vi "Initialize.vi"(8 "error in (no error)":errorcluster, 11 "Instrument in":refnum<class "Instrument.lvclass">) -> (0 "error out":errorcluster, 3 "Instrument out":refnum<class "Instrument.lvclass">)   [LabVIEW 2018, in "Instrument.lvclass"]
uses:
  Instrument.lvclass
  C:/Users/observer/Desktop/Sparc4GUI/SPARC4_GUI/Server/Server.lvclass
  Server/Server.lvclass/Server.ctl
  Instrument.lvclass/Instrument.ctl
  Device/Optics/Optics.lvclass/Optics.ctl
  Device/Optics/Opt_Selector/Opt_Selector.lvclass
  C:/Users/observer/Desktop/Sparc4GUI/SPARC4_GUI/Device/Optics/Optics.lvclass
  Device/Optics/Opt_Continuous/Opt_Continuous.lvclass
  Server/Server.lvclass
  Comm/Stream/Stream.lvclass
  Log/Log.lvclass
  StateMachine/State Machine.lvclass
  Device/Optics/Optics.lvclass
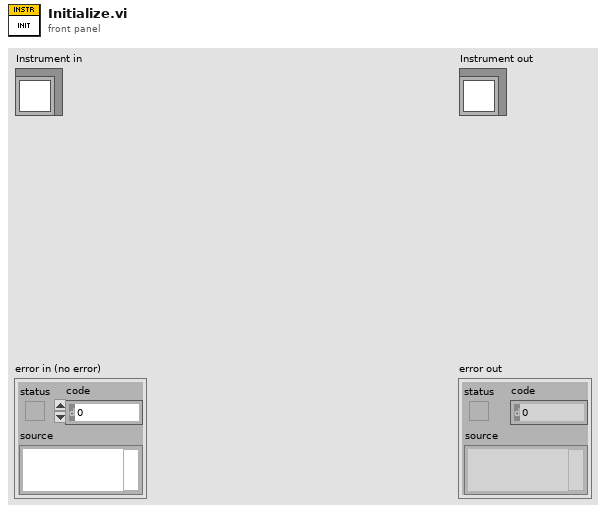
[diagram p1: front panel]
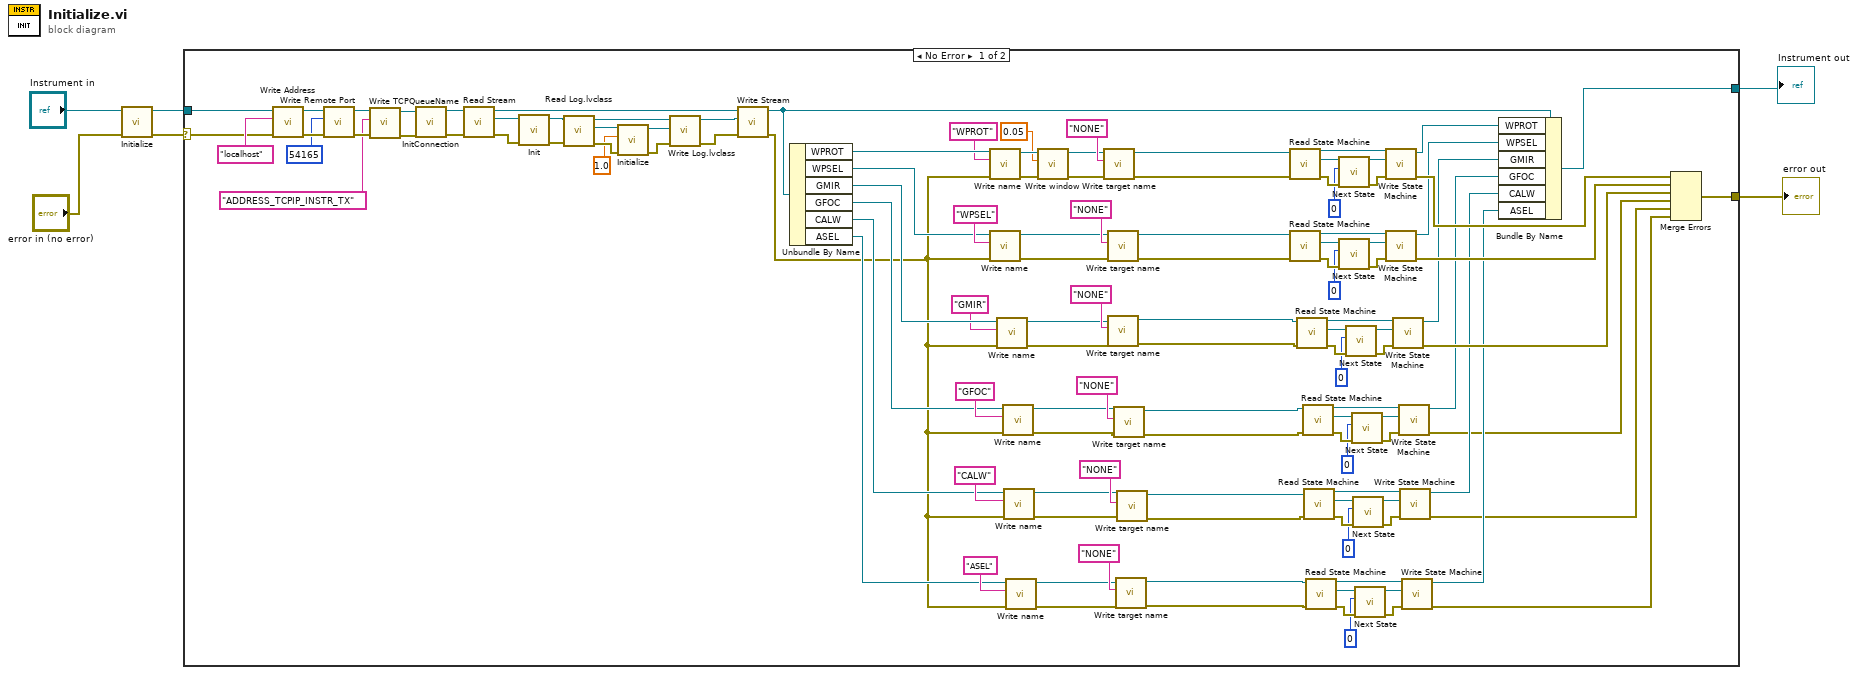
[diagram p0: block diagram]
diagram:
  n1 = call-parent "Initialize.vi"("error in (no error)"="error in (no error)", "Server in"="Instrument in") -> ("error out"=w3:errorcluster, "Server out"=w4:refnum<class "Instrument.lvclass">)  [unwired: 8 in]
  n2 = case shown="No Error" w3 {
    selector: w3 -> [w89 w131]
    tunnel: [w52 w130] -> w1
    tunnel: w4 -> [w90 w130]
    tunnel: [w109 w131] -> w2
    frame No Error {
      n3 = call "Write Address.vi"("error in (no error)"=w89, "Address"="localhost" ("Address:"), "Server in"=w90) -> ("error out"=w93:errorcluster, "Server out"=w94:refnum<class "Instrument.lvclass">)  [unwired: 7 in]
      n4 = call "Write Remote Port.vi"("error in (no error)"=w93, "Remote Port"=u32 54165 ("Remote Port:"), "Server in"=w94) -> ("error out"=w19:errorcluster, "Server out"=w21:refnum<class "Instrument.lvclass">)  [unwired: 7 in]
      n5 = call-dynamic "Write TCPQueueName.vi"("error in (no error)"=w19, "TCPQueueName"="ADDRESS_TCPIP_INSTR_TX", "Server in"=w21) -> ("error out"=w18:errorcluster, "Server out"=w20:refnum<class "Instrument.lvclass">)  [unwired: 7 in]
      n6 = call-dynamic "InitConnection.vi"("error in (no error)"=w18, "Instrument in"=w20) -> ("error out"=w96:errorcluster, "Instrument out"=w95:refnum<class "Instrument.lvclass">)  [unwired: 8 in]
      n7 = call-dynamic "Read Stream.vi"("error in (no error)"=w96, "Server in"=w95) -> ("error out"=w128:errorcluster, "Stream.lvclass"=w53:refnum<class "Stream.lvclass">, "Server out"=w129:refnum<class "Instrument.lvclass">)  [unwired: 7 in]
      n8 = call-dynamic "Init.vi"("error in (no error)"=w128, "Stream in"=w53) -> ("error out"=w10:errorcluster, "Stream out"=w11:refnum<class "Stream.lvclass">)  [unwired: 8 in]
      n9 = call-dynamic "Read Log.lvclass.vi"("error in (no error)"=w10, "Comm in"=w11) -> ("error out"=w13:errorcluster, "Log.lvclass"=w15:refnum<class "Log.lvclass">, "Comm out"=w16:refnum<class "Stream.lvclass">)  [unwired: 7 in]
      n10 = call-dynamic "Initialize.vi"("error in (no error)"=w13, "Level"=1.0, "Log in"=w15) -> ("error out"=w12:errorcluster, "Log out"=w14:refnum<class "Log.lvclass">)  [unwired: 7 in]
      n11 = call-dynamic "Write Log.lvclass.vi"("error in (no error)"=w12, "Log.lvclass"=w14, "Comm in"=w16) -> ("error out"=w8:errorcluster, "Comm out"=w9:refnum<class "Stream.lvclass">)  [unwired: 7 in]
      n12 = call-dynamic "Write Stream.vi"("error in (no error)"=w8, "Stream.lvclass"=w9, "Server in"=w129) -> ("error out"=w63:errorcluster, "Server out"=w54:refnum<class "Instrument.lvclass">)  [unwired: 7 in]
      n13 = Unbundle By Name(w54) -> ("WPROT"=w120:refnum<class "Opt_Selector.lvclass">, "WPSEL"=w111:refnum<class "Opt_Selector.lvclass">, "GMIR"=w100:refnum<class "Opt_Continuous.lvclass">, "GFOC"=w81:refnum<class "Opt_Continuous.lvclass">, "CALW"=w65:refnum<class "Opt_Selector.lvclass">, "ASEL"=w64:refnum<class "Opt_Selector.lvclass">)
      n14 = call-dynamic "Write name.vi"("error in (no error)"=w63, "name"="WPROT", "Optics in"=w120) -> ("error out"=w57:errorcluster, "Optics out"=w56:refnum<class "Opt_Selector.lvclass">)  [unwired: 7 in]
      n15 = call-dynamic "Write name.vi"("error in (no error)"=w63, "name"="WPSEL", "Optics in"=w111) -> ("error out"=w44:errorcluster, "Optics out"=w45:refnum<class "Opt_Selector.lvclass">)  [unwired: 7 in]
      n16 = call-dynamic "Write name.vi"("error in (no error)"=w63, "name"="GMIR", "Optics in"=w100) -> ("error out"=w35:errorcluster, "Optics out"=w37:refnum<class "Opt_Continuous.lvclass">)  [unwired: 7 in]
      n17 = call-dynamic "Write name.vi"("error in (no error)"=w63, "name"="GFOC", "Optics in"=w81) -> ("error out"=w31:errorcluster, "Optics out"=w33:refnum<class "Opt_Continuous.lvclass">)  [unwired: 7 in]
      n18 = call-dynamic "Write name.vi"("error in (no error)"=w63, "name"="CALW", "Optics in"=w65) -> ("error out"=w27:errorcluster, "Optics out"=w29:refnum<class "Opt_Selector.lvclass">)  [unwired: 7 in]
      n19 = call-dynamic "Write name.vi"("error in (no error)"=w63, "name"="ASEL", "Optics in"=w64) -> ("error out"=w23:errorcluster, "Optics out"=w25:refnum<class "Opt_Selector.lvclass">)  [unwired: 7 in]
      n20 = call "Write window.vi"("error in (no error)"=w57, "window"=0.05, "Optics in"=w56) -> ("error out"=w48:errorcluster, "Optics out"=w50:refnum<class "Opt_Selector.lvclass">)  [unwired: 7 in]
      n21 = call "Write target name.vi"("error in (no error)"=w48, "target name"="NONE", "Optics in"=w50) -> ("error out"=w47:errorcluster, "Optics out"=w49:refnum<class "Opt_Selector.lvclass">)  [unwired: 7 in]
      n22 = call "Write target name.vi"("error in (no error)"=w44, "target name"="NONE", "Optics in"=w45) -> ("error out"=w43:errorcluster, "Optics out"=w42:refnum<class "Opt_Selector.lvclass">)  [unwired: 7 in]
      n23 = call "Write target name.vi"("error in (no error)"=w35, "target name"="NONE", "Optics in"=w37) -> ("error out"=w34:errorcluster, "Optics out"=w36:refnum<class "Opt_Continuous.lvclass">)  [unwired: 7 in]
      n24 = call "Write target name.vi"("error in (no error)"=w31, "target name"="NONE", "Optics in"=w33) -> ("error out"=w30:errorcluster, "Optics out"=w32:refnum<class "Opt_Continuous.lvclass">)  [unwired: 7 in]
      n25 = call "Write target name.vi"("error in (no error)"=w23, "target name"="NONE", "Optics in"=w25) -> ("error out"=w22:errorcluster, "Optics out"=w24:refnum<class "Opt_Selector.lvclass">)  [unwired: 7 in]
      n26 = call "Write target name.vi"("error in (no error)"=w27, "target name"="NONE", "Optics in"=w29) -> ("error out"=w26:errorcluster, "Optics out"=w28:refnum<class "Opt_Selector.lvclass">)  [unwired: 7 in]
      n27 = call-dynamic "Read State Machine.vi"("error in (no error)"=w47, "Device in"=w49) -> ("error out"=w124:errorcluster, "State Machine.lvclass"=w127:refnum<class "State Machine.lvclass">, "Device out"=w126:refnum<class "Opt_Selector.lvclass">)  [unwired: 7 in]
      n28 = call-dynamic "Read State Machine.vi"("error in (no error)"=w43, "Device in"=w42) -> ("error out"=w115:errorcluster, "State Machine.lvclass"=w118:refnum<class "State Machine.lvclass">, "Device out"=w117:refnum<class "Opt_Selector.lvclass">)  [unwired: 7 in]
      n29 = call-dynamic "Read State Machine.vi"("error in (no error)"=w34, "Device in"=w36) -> ("error out"=w103:errorcluster, "State Machine.lvclass"=w106:refnum<class "State Machine.lvclass">, "Device out"=w105:refnum<class "Opt_Continuous.lvclass">)  [unwired: 7 in]
      n30 = call-dynamic "Read State Machine.vi"("error in (no error)"=w30, "Device in"=w32) -> ("error out"=w85:errorcluster, "State Machine.lvclass"=w88:refnum<class "State Machine.lvclass">, "Device out"=w87:refnum<class "Opt_Continuous.lvclass">)  [unwired: 7 in]
      n31 = call-dynamic "Read State Machine.vi"("error in (no error)"=w26, "Device in"=w28) -> ("error out"=w76:errorcluster, "State Machine.lvclass"=w79:refnum<class "State Machine.lvclass">, "Device out"=w78:refnum<class "Opt_Selector.lvclass">)  [unwired: 7 in]
      n32 = call-dynamic "Read State Machine.vi"("error in (no error)"=w22, "Device in"=w24) -> ("error out"=w69:errorcluster, "State Machine.lvclass"=w72:refnum<class "State Machine.lvclass">, "Device out"=w71:refnum<class "Opt_Selector.lvclass">)  [unwired: 7 in]
      n33 = call "Next State.vi"("error in (no error)"=w124, "New_State"=0, "State Machine in"=w127) -> ("error out"=w123:errorcluster, "State Machine out"=w125:refnum<class "State Machine.lvclass">)  [unwired: 7 in]
      n34 = call "Next State.vi"("error in (no error)"=w115, "New_State"=0, "State Machine in"=w118) -> ("error out"=w114:errorcluster, "State Machine out"=w116:refnum<class "State Machine.lvclass">)  [unwired: 7 in]
      n35 = call "Next State.vi"("error in (no error)"=w103, "New_State"=0, "State Machine in"=w106) -> ("error out"=w102:errorcluster, "State Machine out"=w104:refnum<class "State Machine.lvclass">)  [unwired: 7 in]
      n36 = call "Next State.vi"("error in (no error)"=w85, "New_State"=0, "State Machine in"=w88) -> ("error out"=w84:errorcluster, "State Machine out"=w86:refnum<class "State Machine.lvclass">)  [unwired: 7 in]
      n37 = call "Next State.vi"("error in (no error)"=w76, "New_State"=0, "State Machine in"=w79) -> ("error out"=w75:errorcluster, "State Machine out"=w77:refnum<class "State Machine.lvclass">)  [unwired: 7 in]
      n38 = call "Next State.vi"("error in (no error)"=w69, "New_State"=0, "State Machine in"=w72) -> ("error out"=w68:errorcluster, "State Machine out"=w70:refnum<class "State Machine.lvclass">)  [unwired: 7 in]
      n39 = call-dynamic "Write State Machine.vi"("error in (no error)"=w123, "State Machine.lvclass"=w125, "Device in"=w126) -> ("error out"=w110:errorcluster, "Device out"=w121:refnum<class "Opt_Selector.lvclass">)  [unwired: 7 in]
      n40 = call-dynamic "Write State Machine.vi"("error in (no error)"=w114, "State Machine.lvclass"=w116, "Device in"=w117) -> ("error out"=w108:errorcluster, "Device out"=w107:refnum<class "Opt_Selector.lvclass">)  [unwired: 7 in]
      n41 = call-dynamic "Write State Machine.vi"("error in (no error)"=w102, "State Machine.lvclass"=w104, "Device in"=w105) -> ("error out"=w98:errorcluster, "Device out"=w99:refnum<class "Opt_Continuous.lvclass">)  [unwired: 7 in]
      n42 = call-dynamic "Write State Machine.vi"("error in (no error)"=w84, "State Machine.lvclass"=w86, "Device in"=w87) -> ("error out"=w58:errorcluster, "Device out"=w80:refnum<class "Opt_Continuous.lvclass">)  [unwired: 7 in]
      n43 = call-dynamic "Write State Machine.vi"("error in (no error)"=w75, "State Machine.lvclass"=w77, "Device in"=w78) -> ("error out"=w60:errorcluster, "Device out"=w62:refnum<class "Opt_Selector.lvclass">)  [unwired: 7 in]
      n44 = call-dynamic "Write State Machine.vi"("error in (no error)"=w68, "State Machine.lvclass"=w70, "Device in"=w71) -> ("error out"=w59:errorcluster, "Device out"=w61:refnum<class "Opt_Selector.lvclass">)  [unwired: 7 in]
      n45 = Bundle By Name(cluster=w54, "WPROT"=w121, "WPSEL"=w107, "GMIR"=w99, "GFOC"=w80, "CALW"=w62, "ASEL"=w61) -> (w52:refnum<class "Instrument.lvclass">)
      n46 = Merge Errors(w110, w108, w98, w58, w60, w59) -> (w109:errorcluster)
    }
    frame Error {
    }
  }
  "error out" <- w2
  "Instrument out" <- w1
